vi "Add CORS Headers.vi"(8 "error in (no error)":errorcluster, 11 "LabVIEW Web Service Request":refnum<class "Web Request.lvclass">) -> (0 "error out":errorcluster, 3 "LabVIEW Web Service Request out":refnum<class "Web Request.lvclass">)   [LabVIEW 2016, in "WSsupport.lvlib"]
uses:
  WSsupport.lvlib
  <vilib>/wsapi/Web Request.lvclass
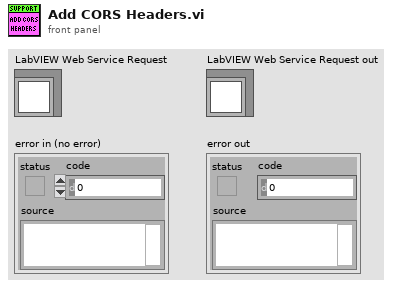
[diagram p1: front panel]
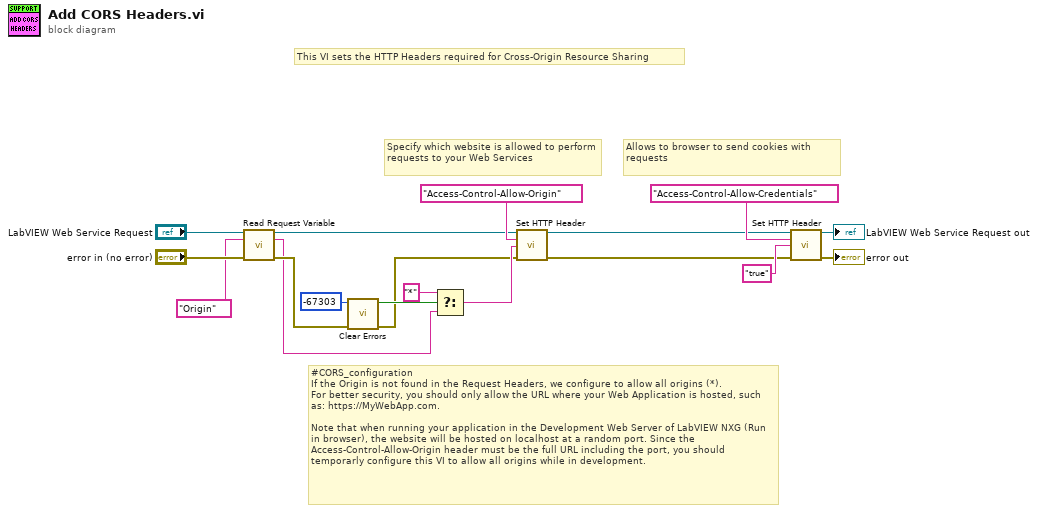
[diagram p0: block diagram]
diagram:
  # "#CORS_configuration\nIf the Origin is not found in the Request Headers, we configure to allow all origins (*).\nFor better security, you should only allow the URL where your Web Application is hosted, such as: https://MyWebApp.com.\n\nNote that when running your application in the Development Web Server of LabVIEW NXG (Run in browser), the website will be hosted on localhost at a random port. Since the Access-Control-Allow-Origin header must be the full URL including the port, you should temporarly configure this VI to allow all origins while in development."
  # "Allows to browser to send cookies with requests"
  # "Specify which website is allowed to perform requests to your Web Services"
  # "This VI sets the HTTP Headers required for Cross-Origin Resource Sharing"
  n1 = call <vilib>:"Read Request Variable.vi"("LabVIEW Web Service Request"="LabVIEW Web Service Request", "variable name"="Origin", "error in (no error)"="error in (no error)") -> ("LabVIEW Web Service Request out"=w6:refnum<class "Web Request.lvclass">, "value"=w8:string, "error out"=w16:errorcluster)  [unwired: 10 in]
  n2 = call <vilib>:"Clear Errors.vi"("error in (no error)"=w16, "specific error code to clear (0: all)"=-67303) -> ("error out"=w4:errorcluster, "specific error cleared?"=w10:bool)  [unwired: 4 in]
  n3 = Select(t="*", s=w10, f=w8) -> (s? t:f=w7:string)
  n4 = call <vilib>:"Set HTTP Header.vi"("LabVIEW Web Service Request"=w6, "header"="Access-Control-Allow-Origin", "header value"=w7, "error in (no error)"=w4) -> ("LabVIEW Web Service Request out"=w5:refnum<class "Web Request.lvclass">, "error out"=w3:errorcluster)  [unwired: 10 in]
  n5 = call <vilib>:"Set HTTP Header.vi"("LabVIEW Web Service Request"=w5, "header"="Access-Control-Allow-Credentials", "header value"="true", "error in (no error)"=w3) -> ("LabVIEW Web Service Request out"=→"LabVIEW Web Service Request out":refnum<class "Web Request.lvclass">, "error out"=→"error out":errorcluster)  [unwired: 10 in]
